vi "Marshall.vi"(8 "error in (no error)":errorcluster, 10 "Variant":variant, 11 "Serializer in":refnum<class "Serializer.lvclass">) -> (0 "error out":errorcluster, 2 "String":string, 3 "Serializer out":refnum<class "Serializer.lvclass">)   [LabVIEW 2013, in "CfgManager.lvlib" / "Serializer.lvclass"]
uses:
  Serializer.lvclass
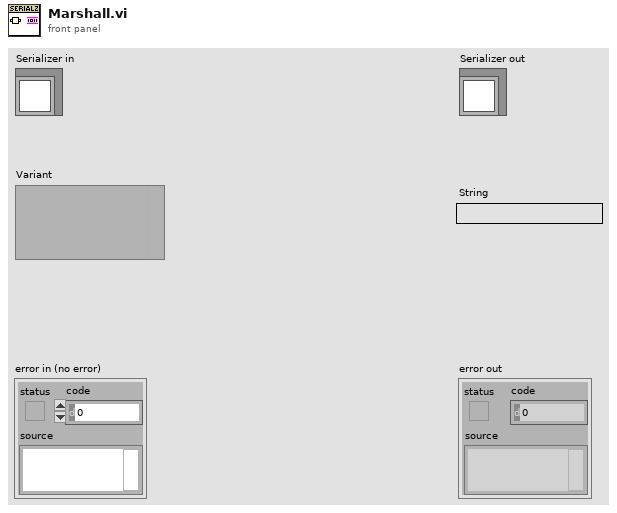
[diagram p1: front panel]
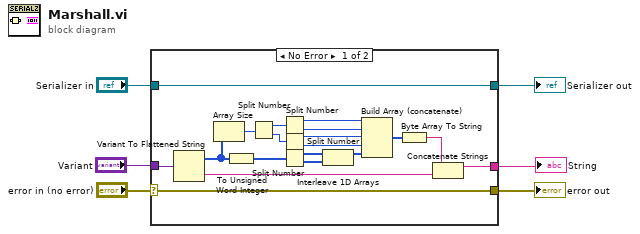
[diagram p0: block diagram]
diagram:
  n1 = case shown="No Error" "error in (no error)" {
    selector: "error in (no error)" -> [w23 w27]
    tunnel: [w23 w27] -> w5
    tunnel: [w25 w26] -> w3
    tunnel: "Serializer in" -> [w25 w26]
    tunnel: "Variant" -> [w22 _]
    tunnel: [w24 _] -> w1
    frame No Error {
      n2 = Variant To Flattened String(Variant=w22) -> (data string=w12:string, 1:w21:i16[])
      n3 = Array Size(array=w21) -> (size(s)=w20:i32)
      n4 = To Unsigned Word Integer(number=w21) -> (unsigned 16bit integer=w11:u16[])
      n5 = Split Number(x=w20) -> (hi(x)=w19:u16, lo(x)=w18:u16)
      n6 = Split Number(x=w19) -> (hi(x)=w17:u8, lo(x)=w16:u8)
      n7 = Split Number(x=w18) -> (hi(x)=w15:u8, lo(x)=w14:u8)
      n8 = Split Number(x=w11) -> (hi(x)=w8:u8[], lo(x)=w9:u8[])
      n9 = Interleave 1D Arrays(w8, w9) -> (w7:u8[])
      n10 = Build Array (concatenate)(w17, w16, w15, w14, w7) -> (w10:u8[])
      n11 = Byte Array To String(unsigned byte array=w10) -> (string=w13:string)
      n12 = Concatenate Strings(w13, w12) -> (w24:string)
    }
    frame Error {
    }
  }
  "error out" <- w5
  "Serializer out" <- w3
  "String" <- w1
